vi "Scale and Download Envelope Waveform.vi"(0 "Envelope Generator Handle in":refnum<k15>, 5 "Envelope Waveform":T1 {"Runtime Scaling" format="%#_6p"; "Sample Rate" format="%#_6p"; "Burst Length (s)" format="%#_6p"; "PAPR (dB)" format="%.2f"; "Signal Bandwidth (Hz)" format="%#_6p"}, 7 "Tracker Configuration":T2={"Input Impedance (Ohms)"=1000000.0, "Common Mode Offset (V)"=1.0, "Gain (V/V)"=2.5, "Output Offset (V)"=2.55} {"Input Impedance (Ohms)" format="%#_6p"}, 11 "error in (no error)":errorcluster) -> (4 "Envelope Generator Handle out":refnum<k15>, 6 "Scaled Envelope Waveform":T1 {"Runtime Scaling" format="%#_6p"; "Sample Rate" format="%#_6p"; "Burst Length (s)" format="%#_6p"; "PAPR (dB)" format="%.2f"; "Signal Bandwidth (Hz)" format="%#_6p"}, 15 "error out":errorcluster)   [LabVIEW 2019, in "Envelope Tracking.lvlib"]
doc: "Scales the envelope waveform data based on the settings in trackerConfig, and downloads the waveform to the envelope generator."
uses:
  Envelope Tracking.lvlib
  Common/Waveform.ctl
  Typedefs/Tracker Configuration.ctl
  Common/Common.lvlib
  SG/SG.lvlib
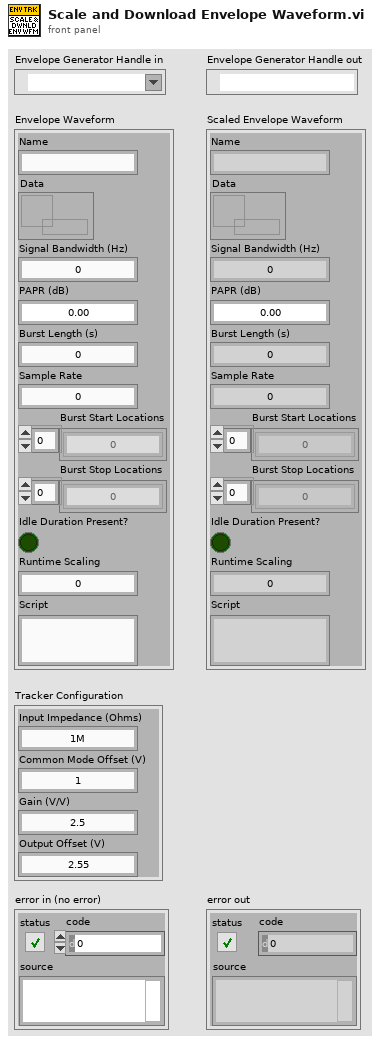
[diagram p1: front panel]
types:
  T1 = typedef "Common.lvlib/Waveform.ctl" = cluster{"Name":string, "Data":refnum<data-value>, "Signal Bandwidth (Hz)":dbl, "PAPR (dB)":dbl, "Burst Length (s)":dbl, "Sample Rate":dbl, "Burst Start Locations":i32[], "Burst Stop Locations":i32[], "Idle Duration Present?":bool, "Runtime Scaling":dbl, "Script":string}
  T2 = typedef "Envelope Tracking.lvlib/Tracker Configuration.ctl" = cluster{"Input Impedance (Ohms)":dbl, "Common Mode Offset (V)":dbl, "Gain (V/V)":dbl, "Output Offset (V)":dbl}
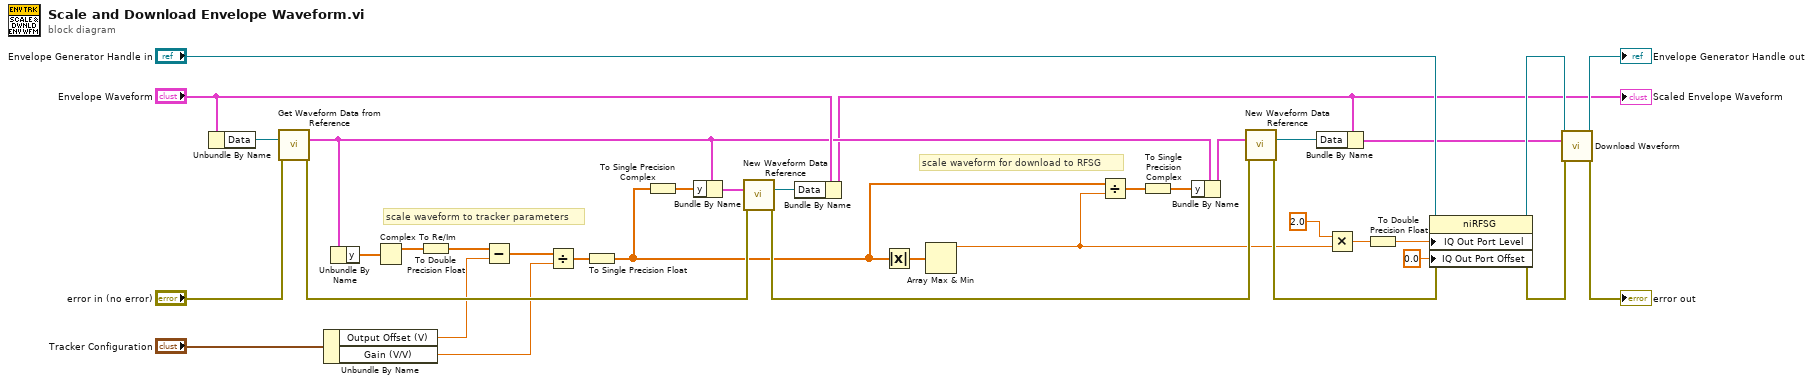
[diagram p0: block diagram]
diagram:
  # "scale waveform for download to RFSG"
  # "scale waveform to tracker parameters"
  n1 = Unbundle By Name("Envelope Waveform") -> ("Data"=w30:refnum<data-value>)
  n2 = call "Get Waveform Data from Reference.vi"("Waveform Data Reference"=w30, "error in (no error)"="error in (no error)") -> ("Waveform Data"=w10:cluster{"t0":dbl, "dt":dbl, "y":csg[]}, "error out"=w35:errorcluster)  [unwired: 12 in]
  n3 = Unbundle By Name("Tracker Configuration") -> ("Output Offset (V)"=w20:dbl, "Gain (V/V)"=w19:dbl)
  n4 = Unbundle By Name(w10) -> ("y"=w29:csg[])
  n5 = Complex To Re/Im(x + iy=w29) -> (x=w27:sgl[])  [unwired: 1 out]
  n6 = To Double Precision Float(number=w27) -> (double precision float=w18:dbl[])
  n7 = Subtract(x=w18, y=w20) -> (x-y=w26:dbl[])
  n8 = Divide(x=w26, y=w19) -> (x/y=w16:dbl[])
  n9 = To Single Precision Float(number=w16) -> (single precision float=w12:sgl[])
  n10 = To Single Precision Complex(1:w12) -> (0:w17:csg[])
  n11 = Bundle By Name(cluster=w10, "y"=w17) -> (w15:cluster{"t0":dbl, "dt":dbl, "y":csg[]})
  n12 = call "New Waveform Data Reference.vi"("Waveform Data"=w15, "error in (no error)"=w35) -> ("Waveform Data Reference"=w14:refnum<data-value>, "error out"=w34:errorcluster)  [unwired: 12 in]
  n13 = Bundle By Name(cluster="Envelope Waveform", "Data"=w14) -> (w6:T1)
  "Scaled Envelope Waveform" <- w6
  n14 = Absolute Value(x=w12) -> (abs(x)=w11:sgl[])
  n15 = Array Max & Min(array=w11) -> (max value=w3:sgl)  [unwired: 3 out]
  n16 = Divide(x=w12, y=w3) -> (x/y=w9:sgl[])
  n17 = To Single Precision Complex(1:w9) -> (0:w8:csg[])
  n18 = Bundle By Name(cluster=w10, "y"=w8) -> (w7:cluster{"t0":dbl, "dt":dbl, "y":csg[]})
  n19 = call "New Waveform Data Reference.vi"("Waveform Data"=w7, "error in (no error)"=w34) -> ("Waveform Data Reference"=w5:refnum<data-value>, "error out"=w33:errorcluster)  [unwired: 12 in]
  n20 = Bundle By Name(cluster=w6, "Data"=w5) -> (w4:T1)
  n21 = Multiply(x=sgl 2.0 ("y"), y=w3) -> (x*y=w1:sgl)
  n22 = To Double Precision Float(number=w1) -> (double precision float=w25:dbl)
  n23 = property class="niRFSG"(reference="Envelope Generator Handle in", error in=w33, "IQ Out Port Level"=w25, "IQ Out Port Offset"=0.0 ("Device Specific:Vector Signal Transceiver:IQ Out Port:Offset")) -> (reference out=w22:refnum<k15>, error out=w32:errorcluster)
  n24 = call "Download Waveform.vi"("RFSG handle"=w22, "Waveform In"=w4, "error in (no error)"=w32) -> ("RFSG handle out"=→"Envelope Generator Handle out":refnum<k15>, "error out"=→"error out":errorcluster)  [unwired: 11 in]
